vi "zad1.vi"() -> ()   [LabVIEW 2025]
panel:
  out "initialized array 2":dbl[](array[numeric])
  out "Array 2":dbl[](array[numeric])
  out "initialized array":dbl[](array[numeric])
  out "Array":dbl[](array[numeric])
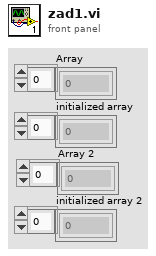
[diagram p1: front panel]
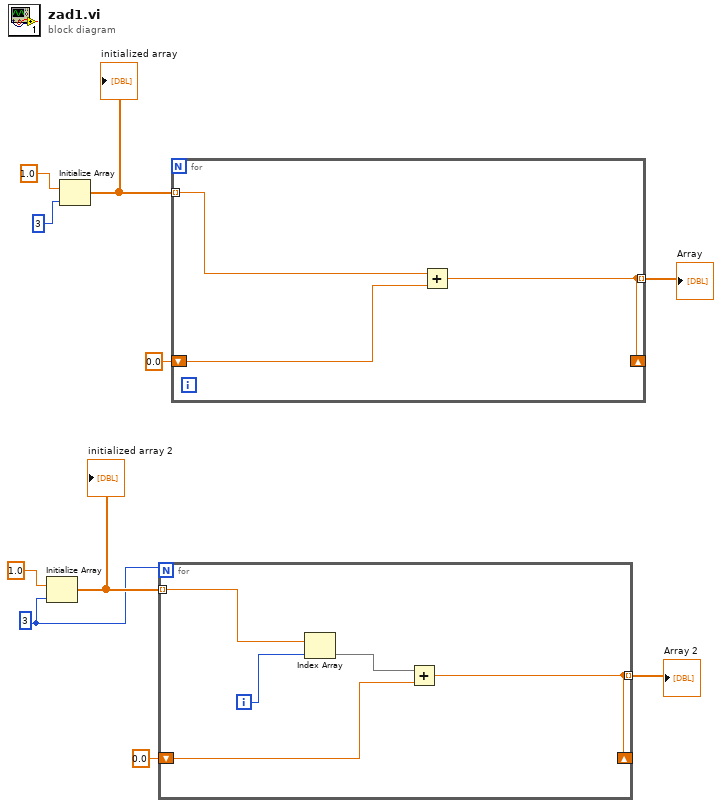
[diagram p0: block diagram]
diagram:
  w1 = 3 ("dimension size")
  n1 = Initialize Array(1.0 ("element"), w1) -> (w4:dbl[])
  "initialized array 2" <- w4
  n2 = Initialize Array(1.0 ("element"), 3 ("dimension size")) -> (w8:dbl[])
  "initialized array" <- w8
  n3 = for {
    N: w1 -> [_]
    shift-right: [w14] -> _
    shift-left: 0.0 -> [w15]
    tunnel: w4 -> [w11] mode=indexing
    tunnel: [w14] -> w2 mode=indexing
    i -> [w12]
    n4 = Index Array(array=w11, index=w12) -> (element=w13)
    n5 = Add(x=w13, y=w15) -> (x+y=w14:dbl)
  }
  "Array 2" <- w2
  n6 = for {
    shift-right: [w16] -> _
    shift-left: 0.0 -> [w18]
    tunnel: w8 -> [w17] mode=indexing
    tunnel: [w16] -> w6 mode=indexing
    n7 = Add(x=w17, y=w18) -> (x+y=w16:dbl)
  }
  "Array" <- w6
